vi "Create GUID Property.vi"(8 "error in (no error)":errorcluster) -> (0 "error out":errorcluster, 2 "property values":string[](array[string]), 3 "property names":string[](array[string]))   [LabVIEW 2018, in "Instrument Addon Scripting API.lvlib"]
uses:
  Instrument Addon Scripting API.lvlib
  Addon/Addon Shared/SubVIs/Constants.vi
  Addon/Addon Shared/Instrument Addon Shared.lvlib
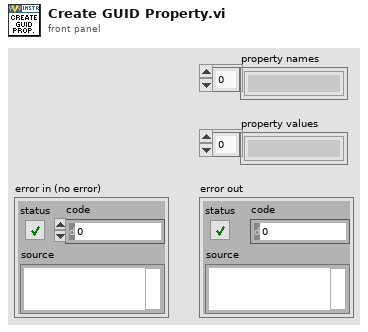
[diagram p1: front panel]
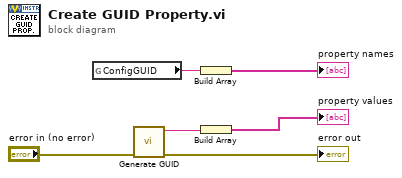
[diagram p0: block diagram]
diagram:
  n1 = global read "Constants.vi" "ConfigGUID"() -> (w3:string)
  n2 = call "Generate GUID.vi"("error in (no error)"="error in (no error)") -> ("error out"=→"error out":errorcluster, "GUID"=w4:string)  [unwired: 9 in]
  n3 = Build Array(w3) -> (→"property names":string[])
  n4 = Build Array(w4) -> (→"property values":string[])
